vi "Write Service.vi"(8 "error in (no error)":errorcluster, 10 "Service":string, 11 "AWS Core in":refnum<class "AWS Core.lvclass">) -> (0 "error out":errorcluster, 3 "AWS Core out":refnum<class "AWS Core.lvclass">)   [LabVIEW 2015, in "AWS Core.lvlib" / "AWS Core.lvclass"]
uses:
  AWS Core.lvclass
  AWS Core.lvclass/AWS Core.ctl
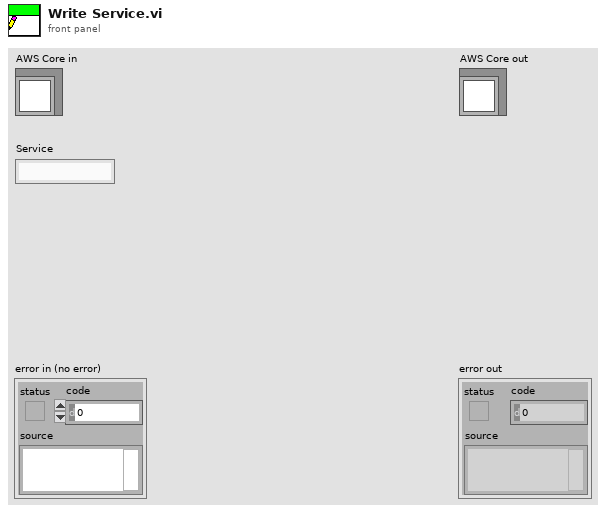
[diagram p1: front panel]
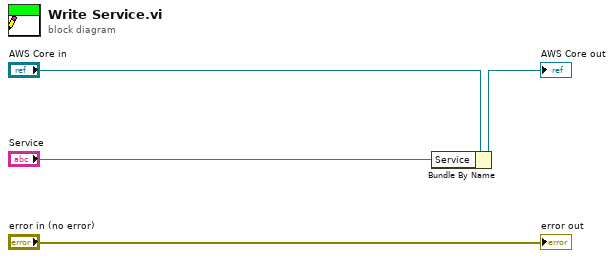
[diagram p0: block diagram]
diagram:
  n1 = Bundle By Name(cluster="AWS Core in", "Service"="Service") -> (→"AWS Core out":refnum<class "AWS Core.lvclass">)
  "error out" <- "error in (no error)"
